vi "Read Triggerable Frames.vi"(8 "error in (no error)":errorcluster, 11 "triggers execution unit":refnum<class "Triggers Execution Unit.lvclass">) -> (0 "error out":errorcluster, 2 "triggerable frames":T1[](array[typedef]) {"Acyclic Messages"."Timestamp Channel Handle" format="%.0x"; "Acyclic Messages"."Message Section Handle" format="%.0x"; "Acyclic Messages"."Parameter Channel Handles" format="%.0x"}, 3 "triggers execution unit out":refnum<class "Triggers Execution Unit.lvclass">)   [LabVIEW 2020, in "AIM MIL-STD-1553 Engine.lvlib" / "Implementation.lvlib" / "Triggers Execution Unit.lvclass"]
uses:
  Triggers Execution Unit.lvclass
  Triggerable Frame.ctl
  Custom Device/Compiled Message.ctl
  <vilib>/NI VeriStand/Custom Device API/Custom Device Item Ref.ctl
  Shared/Direction.ctl
  Shared/Parameter Definition.ctl
  Triggers Execution Unit.lvclass/Triggers Execution Unit.ctl
  <vilib>/NI VeriStand/Custom Device API/Custom Device API.lvlib
  Custom Device/Custom Device.lvlib
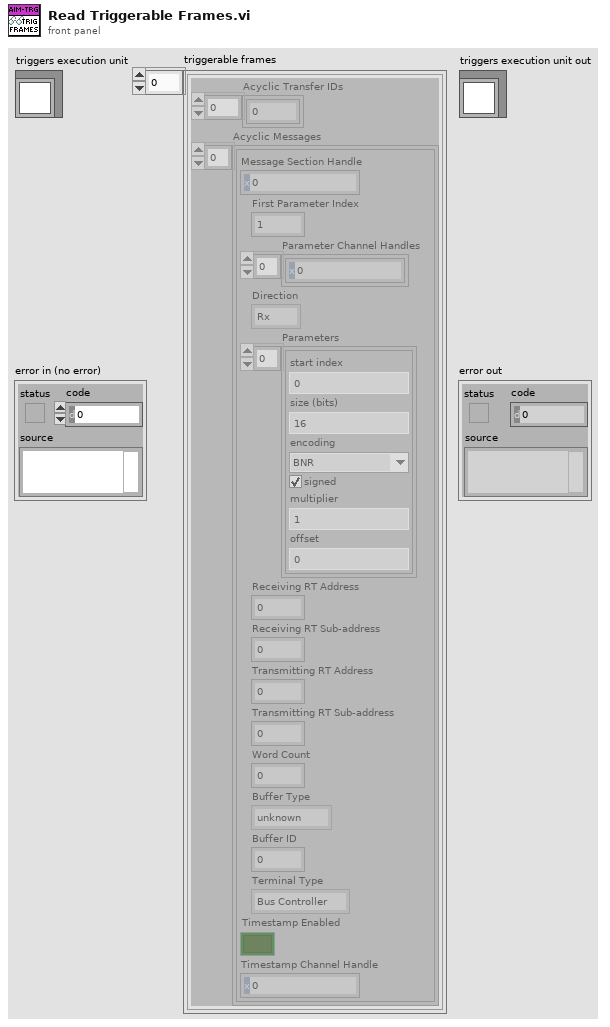
[diagram p1: front panel]
types:
  T1 = typedef "AIM MIL-STD-1553 Engine.lvlib/Implementation.lvlib/Triggers Execution Unit.lvclass/Triggerable Frame.ctl" = cluster{"Acyclic Transfer IDs":u16[], "Acyclic Messages":T2[]}
  T2 = typedef "AIM MIL-STD-1553 Engine.lvlib/Custom Device.lvlib/Compiled Message.ctl" = cluster{"Message Section Handle":T3, "First Parameter Index":i32, "Parameter Channel Handles":T3[], "Direction":T4, "Parameters":T5[], "Receiving RT Address":u8, "Receiving RT Sub-address":u8, "Transmitting RT Address":u8, "Transmitting RT Sub-address":u8, "Word Count":u8, "Buffer Type":enum16{"unknown", "BC Message Buffer", "RT Message Buffer"}, "Buffer ID":u16, "Terminal Type":enum16{"Bus Controller", "Remote Terminal"}, "Timestamp Enabled":bool, "Timestamp Channel Handle":T3}
  T3 = typedef "Custom Device API.lvlib/Custom Device Item Ref.ctl" = u64
  T4 = typedef "Direction.ctl" = enum16{"Rx", "Tx"}
  T5 = typedef "Parameter Definition.ctl" = cluster{"start index":i32, "size (bits)":i32, "encoding":enum16{"BNR", "BCD", "Discrete"}, "signed":bool, "multiplier":dbl, "offset":dbl}
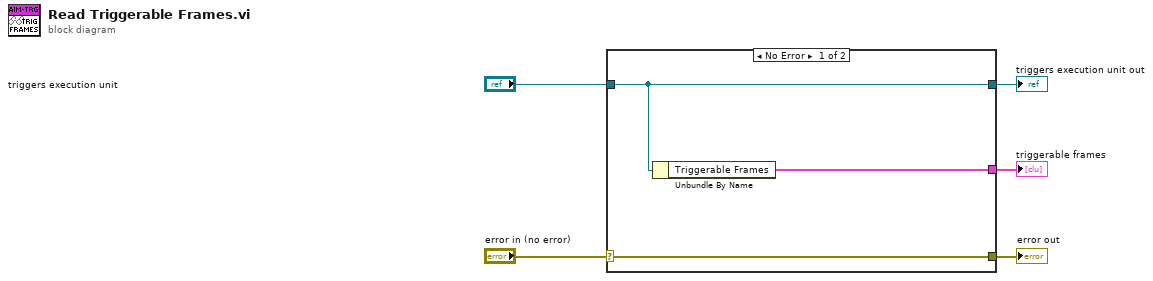
[diagram p0: block diagram]
diagram:
  n1 = case shown="No Error" "error in (no error)" {
    selector: "error in (no error)" -> [w8 w9]
    tunnel: [w8 w9] -> w4
    tunnel: [w7 w10] -> w2
    tunnel: "triggers execution unit" -> [w7 w10]
    tunnel: [w6 _] -> w1
    frame No Error {
      n2 = Unbundle By Name(w7) -> ("Triggerable Frames"=w6:T1[])
    }
    frame Error {
    }
  }
  "error out" <- w4
  "triggers execution unit out" <- w2
  "triggerable frames" <- w1
